vi "Example Command to Main.vi"(8 "error in (no error)":errorcluster, 10 "Command Data":i32, 11 "TemplatePlugin in":refnum<class "Template_Plugin.lvclass">) -> (0 "error out":errorcluster, 3 "TemplatePlugin out":refnum<class "Template_Plugin.lvclass">)   [LabVIEW 2021, in "Template_Plugin.lvclass"]
uses:
  Template_Plugin.lvclass
  Template_Plugin.lvclass/Template_Plugin.ctl
  8779bfbf-2797-4940-8d62-f4162e828731.vi
  Common/Typedef/OOB Comm/To Main Command.ctl
  Common/Template_Common.lvlib
  Common/Typedef/OOB Comm/To Main Command Data.ctl
  Common/Typedef/OOB Comm/To Main Command Payload.ctl
  cb651c69-5256-45bc-b9b0-1818fa9c55ac.vi
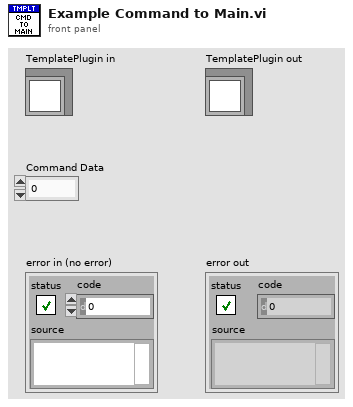
[diagram p1: front panel]
types:
  T1 = typedef "Template_Common.lvlib/To Main Command Payload.ctl" = cluster{"Command":T2, "-> Main":T3}
  T2 = typedef "Template_Common.lvlib/To Main Command.ctl" = enum16{"Read Data", "Read DVR Data"}
  T3 = typedef "Template_Common.lvlib/To Main Command Data.ctl" = cluster{"Cmd Data 1 -> Main":i32}
  T4 = typedef "Template_Common.lvlib/To Main DVR Data.ctl" = cluster{"Data 1 DVR  -> Main":i32}
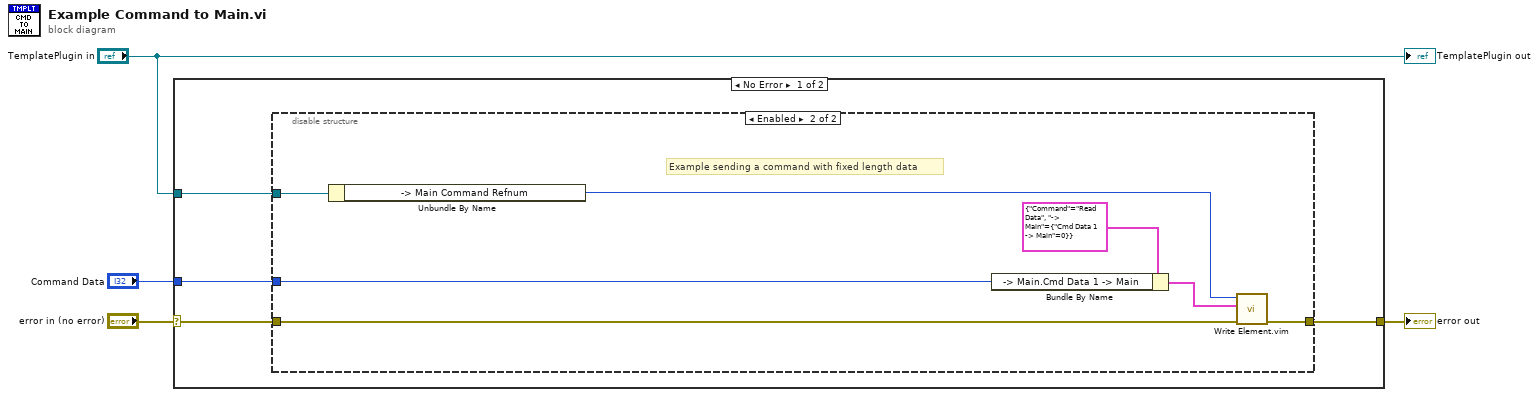
[diagram p0: block diagram]
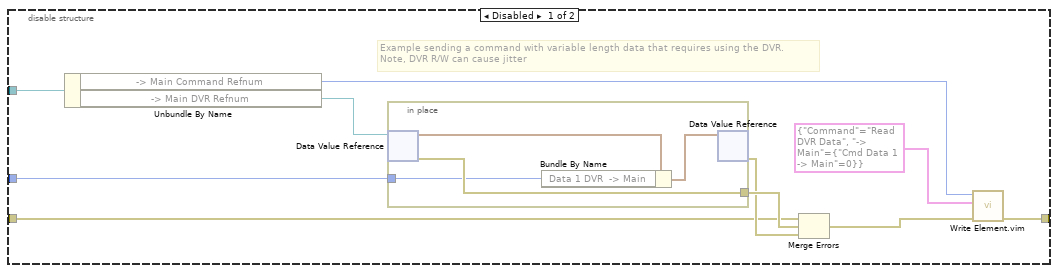
[diagram p2: hidden frame]
diagram:
  n1 = case shown="No Error" "error in (no error)" {
    selector: "error in (no error)" -> [w6 w30]
    tunnel: [w5 w30] -> w3
    tunnel: "TemplatePlugin in" -> [w8 _]
    tunnel: "Command Data" -> [w7 _]
    frame No Error {
      n2 = disable-structure shown="Enabled" {
        disable-tunnel: w8 -> [w13 w28]
        disable-tunnel: w7 -> [w12 w24]
        disable-tunnel: w6 -> [w11 w26]
        disable-tunnel: [w10 w27] -> w5
        frame Disabled {
          # "Example sending a command with variable length data that requires using the DVR.\nNote, DVR R/W can cause jitter"
          n3 = Unbundle By Name(w13) -> ("-> Main Command Refnum"=w15:u64, "-> Main DVR Refnum"=w18:refnum<data-value>)
          n4 = in-place {
            in-place-border: [w20] -> w16
            in-place-border: w12 -> [w19]
            n5 = in-place-dvr #1(w18) -> (w22:T4, w20:errorcluster)
            n6 = Bundle By Name(cluster=w22, "Data 1 DVR  -> Main"=w19) -> (w21:T4)
            n7 = in-place-dvr #1(w21) -> (w14:errorcluster)  [unwired: 1 out]
          }
          n8 = Merge Errors(w11, w16, w14) -> (w17:errorcluster)
          n9 = call "Write Element.vim"("error in (no error)"=w17, "Data in"=T1 {"Command"=enum."Read DVR Data", "-> Main"={"Cmd Data 1 -> Main"=0}} ("Payload"), "CIPC Reference in"=w15) -> ("error out"=w10:errorcluster)  [unwired: 5 in, 3 out]
        }
        frame Enabled {
          # "Example sending a command with fixed length data"
          n10 = Unbundle By Name(w28) -> ("-> Main Command Refnum"=w29:u64)
          n11 = Bundle By Name(cluster=T1 {"Command"=enum."Read Data", "-> Main"={"Cmd Data 1 -> Main"=0}} ("Payload"), "-> Main.Cmd Data 1 -> Main"=w24) -> (w23:T1)
          n12 = call "Write Element.vim"("error in (no error)"=w26, "Data in"=w23, "CIPC Reference in"=w29) -> ("error out"=w27:errorcluster)  [unwired: 5 in, 3 out]
        }
      }
    }
    frame Error {
    }
  }
  "error out" <- w3
  "TemplatePlugin out" <- "TemplatePlugin in"
